vi "FTW-Test-JSON-ObjectJoin.vi"() -> (0 "Test Result":errorcluster)   [LabVIEW 2014]
uses:
  src/core/json/FTW-JSON-UpdateMode.ctl
  src/core/error/FTW-ERR-Assert-DeveloperError.vi
  src/core/error/FTW-ERR-ThrowError.vi
  src/core/error/FTW-ERR-CallChain.vi
  src/core/string/FTW-STR-ReplaceWhitespace.vi
panel:
  out "Joined Objects":string[](array[string])
  out "JSON to Join":string
  out "Original JSON":string
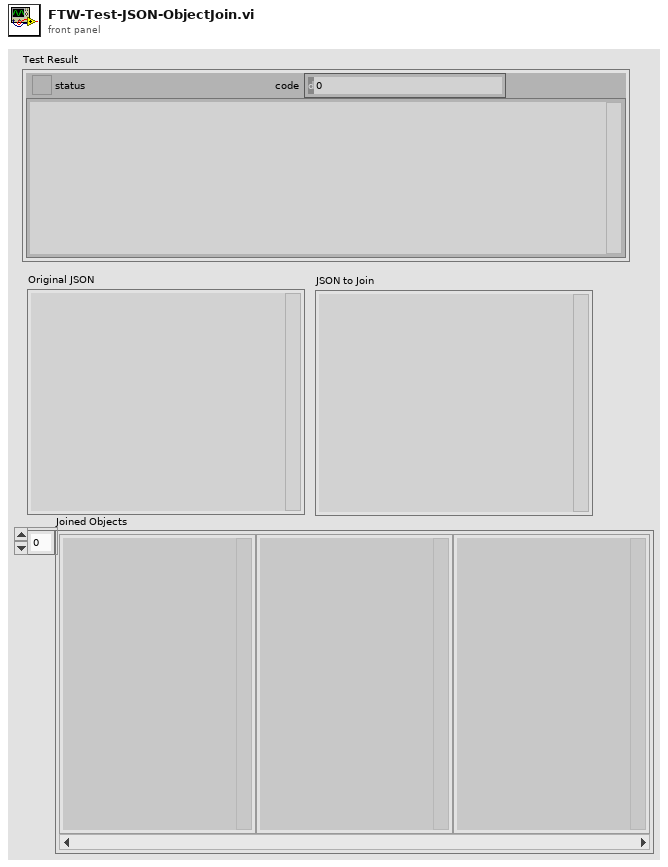
[diagram p1: front panel]
types:
  T1 = typedef "FTW-JSON-UpdateMode.ctl" = enum32{"Upsert", "Update Only", "Insert Only"}
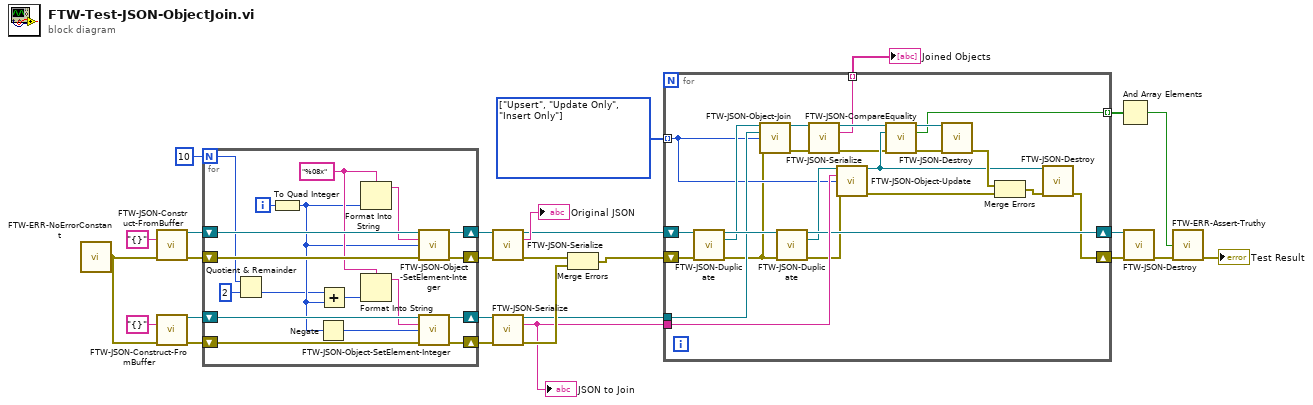
[diagram p0: block diagram]
diagram:
  w9 = T1[] [enum."Upsert", enum."Update Only", enum."Insert Only"] items=["Upsert", "Update Only", "Insert Only"]
  n1 = call "FTW-ERR-NoErrorConstant.vi"() -> ("no error"=w18:errorcluster)
  n2 = call "FTW-JSON-Construct-FromBuffer.vi"("JSON String (UTF-8)"="{}", "error in"=w18) -> ("JSON Object"=w21:refnum<data-value>, "error out"=w20:errorcluster)  [unwired: 12 in]
  n3 = call "FTW-JSON-Construct-FromBuffer.vi"("JSON String (UTF-8)"="{}", "error in"=w18) -> ("JSON Object"=w16:refnum<data-value>, "error out"=w17:errorcluster)  [unwired: 12 in]
  n4 = for {
    N: 10 -> [w30]
    shift-right: [w41] -> w23
    shift-left: w20 -> [w43]
    shift-right: [w44] -> w24
    shift-left: w21 -> [w45]
    shift-right: [w36] -> w14
    shift-left: w17 -> [w38]
    shift-right: [w37] -> w15
    shift-left: w16 -> [w39]
    i -> [w40]
    w35 = "%08x" ("format string")
    n5 = Quotient & Remainder(x=w30, y=2) -> (floor(x/y)=w28:i32)  [unwired: 1 out]
    n6 = To Quad Integer(1:w40) -> (0:w32:i64)
    n7 = Negate(x=w32) -> (-x=w33:i64)
    n8 = Add(x=w28, y=w32) -> (x+y=w31:i64)
    n9 = Format Into String(format string=w35, w32) -> (resulting string=w42:string)  [unwired: 2 in, 1 out]
    n10 = Format Into String(format string=w35, w31) -> (resulting string=w34:string)  [unwired: 2 in, 1 out]
    n11 = call "FTW-JSON-Object-SetElement-Integer.vi"("JSON Object"=w45, "Key"=w42, "Value"=w32, "error in"=w43) -> ("JSON Object out"=w44:refnum<data-value>, "error out"=w41:errorcluster)  [unwired: 10 in]
    n12 = call "FTW-JSON-Object-SetElement-Integer.vi"("JSON Object"=w39, "Key"=w34, "Value"=w33, "error in"=w38) -> ("JSON Object out"=w37:refnum<data-value>, "error out"=w36:errorcluster)  [unwired: 10 in]
  }
  n13 = call "FTW-JSON-Serialize.vi"("JSON Object"=w24, "error in"=w23) -> ("JSON Object out"=w13:refnum<data-value>, "JSON String (UTF-8)"=→"Original JSON":string, "error out"=w11:errorcluster)  [unwired: 11 in]
  n14 = call "FTW-JSON-Serialize.vi"("JSON Object"=w15, "error in"=w14) -> ("JSON Object out"=w8:refnum<data-value>, "JSON String (UTF-8)"=w7:string, "error out"=w12:errorcluster)  [unwired: 11 in]
  "JSON to Join" <- w7
  n15 = Merge Errors(w11, w12) -> (w10:errorcluster)
  n16 = for {
    tunnel: w9 -> [w55] mode=indexing
    tunnel: w8 -> [w64]
    tunnel: w7 -> [w66]
    shift-right: [w63] -> w6
    shift-left: w13 -> [w69]
    tunnel: [w62] -> w3 mode=indexing
    shift-right: [w58] -> w5
    shift-left: w10 -> [w67]
    tunnel: [w50] -> w4 mode=indexing
    n17 = call "FTW-JSON-Duplicate.vi"("JSON Object"=w69, "error in"=w67) -> ("JSON Object out"=w68:refnum<data-value>, "Duplicated JSON Object"=w57:refnum<data-value>, "error out"=w48:errorcluster)  [unwired: 11 in]
    n18 = call "FTW-JSON-Object-Join.vi"("JSON Object"=w57, "JSON Object to Merge"=w64, "Join Mode"=w55, "error in"=w48) -> ("JSON Object out"=w53:refnum<data-value>, "error out"=w49:errorcluster)  [unwired: 10 in]
    n19 = call "FTW-JSON-Duplicate.vi"("JSON Object"=w68, "error in"=w48) -> ("JSON Object out"=w63:refnum<data-value>, "Duplicated JSON Object"=w56:refnum<data-value>, "error out"=w54:errorcluster)  [unwired: 11 in]
    n20 = call "FTW-JSON-Serialize.vi"("JSON Object"=w53, "error in"=w49) -> ("JSON Object out"=w52:refnum<data-value>, "JSON String (UTF-8)"=w50:string, "error out"=w46:errorcluster)  [unwired: 11 in]
    n21 = call "FTW-JSON-Object-Update.vi"("JSON Object"=w56, "JSON Object to Merge"=w66, "Update Mode"=w55, "error in"=w54) -> ("JSON Object out"=w51:refnum<data-value>, "error out"=w47:errorcluster)  [unwired: 10 in]
    n22 = call "FTW-JSON-CompareEquality.vi"("JSON Object"=w52, "JSON Object to Compare"=w51, "error in"=w46) -> ("JSON Object out"=w65:refnum<data-value>, "Equal?"=w62:bool, "error out"=w61:errorcluster)  [unwired: 10 in]
    n23 = call "FTW-JSON-Destroy.vi"("JSON Object"=w65, "error in"=w61) -> ("error out"=w60:errorcluster)  [unwired: 13 in]
    n24 = Merge Errors(w60, w47) -> (w59:errorcluster)
    n25 = call "FTW-JSON-Destroy.vi"("JSON Object"=w51, "error in"=w59) -> ("error out"=w58:errorcluster)  [unwired: 13 in]
  }
  "Joined Objects" <- w4
  n26 = And Array Elements(Boolean array=w3) -> (logical AND=w2:bool)
  n27 = call "FTW-JSON-Destroy.vi"("JSON Object"=w6, "error in"=w5) -> ("error out"=w1:errorcluster)  [unwired: 13 in]
  n28 = call "FTW-ERR-Assert-Truthy.vi"("Expected Truthy"=w2, "error in"=w1) -> ("error out"=→"Test Result":errorcluster)  [unwired: 13 in]
